vi "Obtain-FAMM-Queue.vi"() -> (6 "FAMM-Queue":refnum<queue>)   [LabVIEW 2020]
doc: "Obtain a queue for FAMM service"
uses:
  controls/typedef_FAMM_Query.ctl
  controls/typedef-functions.ctl
  Builds/Sgraph_lib_V1.lvlib
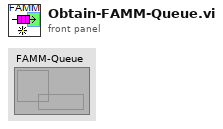
[diagram p1: front panel]
types:
  T1 = typedef "typedef_FAMM_Query.ctl" = cluster{"Time Stamp":timestamp, "FAMM-function":T2, "Source":string, "Data":variant}
  T2 = typedef "Sgraph_lib_V1.lvlib/typedef-functions.ctl" = enum16{"PAQ-request", "PAQ-taglist-request", "WAQ-request", "EAQ-request", "TAG-based-request", "PAQ-MemoryMap", "Update-TAG-property", "Exit-FAMM"}
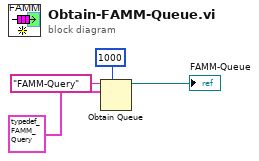
[diagram p0: block diagram]
diagram:
  n1 = Obtain Queue(max queue size (-1, unlimited)=1000, name (unnamed)="FAMM-Query", element data type=T1 {"Time Stamp"=timestamp(0 s since 1904-01-01), "FAMM-function"=enum."PAQ-request", "Source"="", "Data"=variant(dbl[] [])} ("DAQ")) -> (queue out=→"FAMM-Queue":refnum<queue>)  [unwired: 2 in, 2 out]
